vi "Экран наладки.vi"() -> ()   [LabVIEW 2011]
panel:
  in  "Закрыть окно":bool
  in  "y0":dbl
  in  "x40":dbl
  out "y0":bool[](array[boolean])
  out "y0":string[](array[string])
  out "x40":bool[](array[boolean])
  out "x40":string[](array[string])
  out "x0":bool[](array[boolean])
  out "x0":string[](array[string])
  in  "x0":dbl
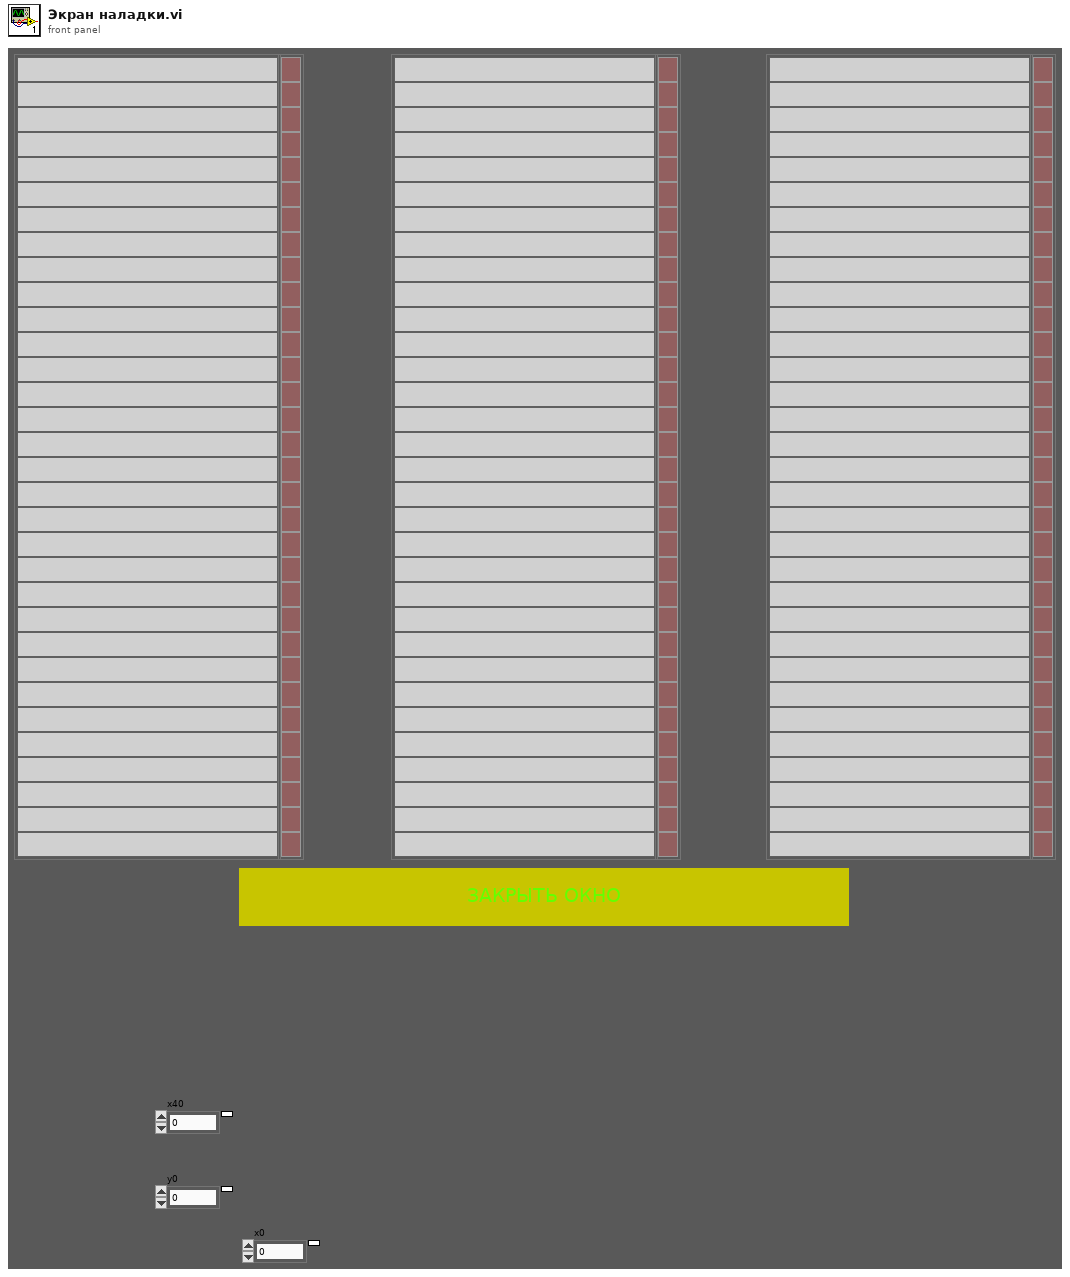
[diagram p1: front panel]
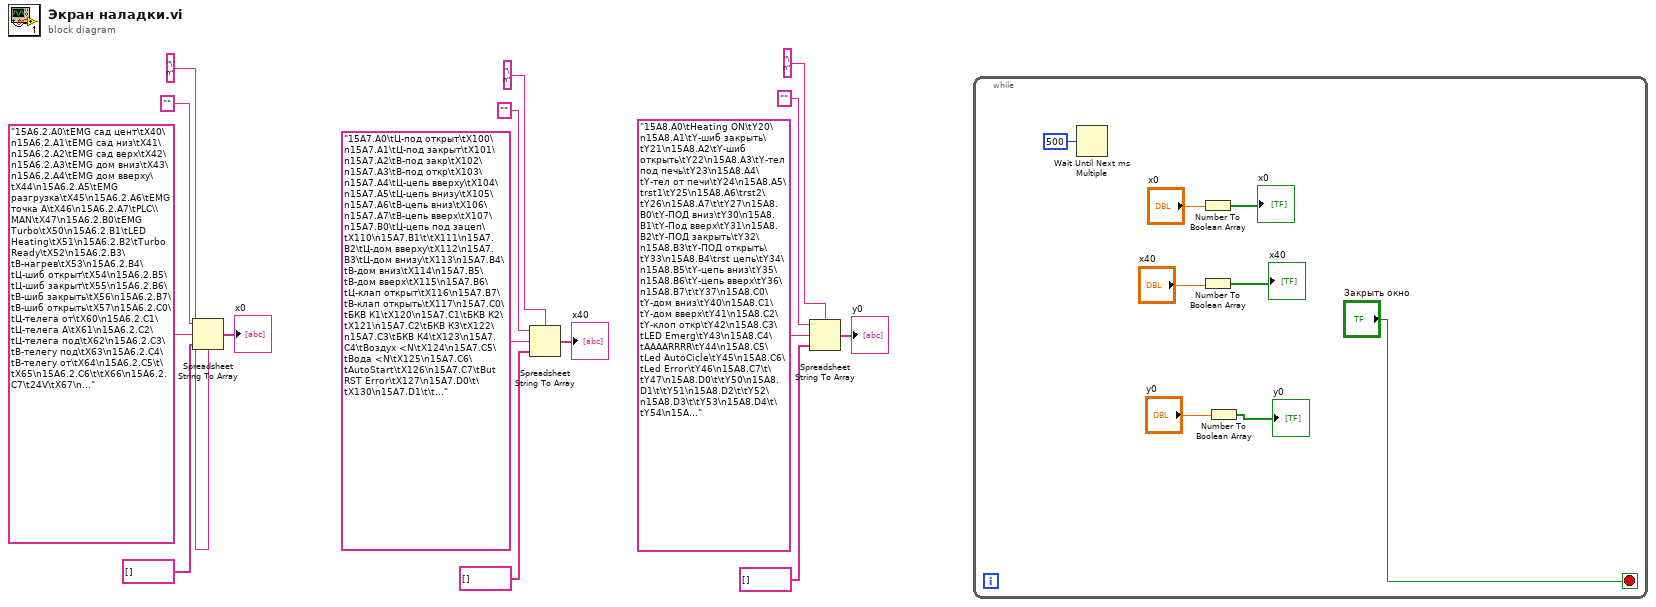
[diagram p0: block diagram]
diagram:
  n1 = Spreadsheet String To Array(delimiter (Tab)="\n", format string="", spreadsheet string="15A6.2.A0\tEMG сад цент\tX40\n15A6.2.A1\tEMG сад низ\tX41\n15A6.2.A2\tEMG сад верх\tX42\n15A6.2.A3\tEMG дом вниз\tX43\n15A6.2.A4\tEMG дом вверху\tX44\n15A6.2.A5\tEMG разгрузка\tX45\n15A6.2.A6\tEMG точка А\tX46\n15A6.2.A7\tPLC\\MAN\tX47\n15A6.2.B0\tEMG Turbo\tX50\n15A6.2.B1\tLED Heating\tX51\n15A6.2.B2\tTurbo Ready\tX52\n15A6.2.B3\tB-нагрев\tX53\n15A6.2.B4\tЦ-шиб открыт\tX54\n15A6.2.B5\tЦ-шиб закрыт\tX55\n15A6.2.B6\tВ-шиб закрыть\tX56\n15A6.2.B7\tВ-шиб открыть\tX57\n15A6.2.C0\tЦ-телега от\tX60\n15A6.2.C1\tЦ-телега А\tX61\n15A6.2.C2\tЦ-телега под\tX62\n15A6.2.C3\tВ-телегу под\tX63\n15A6.2.C4\tВ-телегу от\tX64\n15A6.2.C5\t\tX65\n15A6.2.C6\t\tX66\n15A6.2.C7\t24V\tX67\n15A6.2.D0\tЦ-под up\tX70\n15A6.2.D1\tЦ-под down\tX71\n15A6.2.D2\tВ-под вниз\tX72\n15A6.2.D3\tВ-под вверх\tX73\n15A6.2.D4\tЦ-под2 вверху\tX74\n15A6.2.D5\tЦ-под2 внизу\tX75\n15A6.2.D6\t\tX76\n15A6.2.D7\t\tX77", array type (2D Dbl)=string[] []) -> (array=→"x0":string[])
  n2 = Spreadsheet String To Array(delimiter (Tab)="\n", format string="", spreadsheet string="15A7.A0\tЦ-под открыт\tX100\n15A7.A1\tЦ-под закрыт\tX101\n15A7.A2\tВ-под закр\tX102\n15A7.A3\tВ-под откр\tX103\n15A7.A4\tЦ-цепь вверху\tX104\n15A7.A5\tЦ-цепь внизу\tX105\n15A7.A6\tВ-цепь вниз\tX106\n15A7.A7\tВ-цепь вверх\tX107\n15A7.B0\tЦ-цепь под зацеп\tX110\n15A7.B1\t\tX111\n15A7.B2\tЦ-дом вверху\tX112\n15A7.B3\tЦ-дом внизу\tX113\n15A7.B4\tВ-дом вниз\tX114\n15A7.B5\tВ-дом вверх\tX115\n15A7.B6\tЦ-клап открыт\tX116\n15A7.B7\tВ-клап открыть\tX117\n15A7.C0\tБКВ К1\tX120\n15A7.C1\tБКВ К2\tX121\n15A7.C2\tБКВ К3\tX122\n15A7.C3\tБКВ К4\tX123\n15A7.C4\tВоздух <N\tX124\n15A7.C5\tВода <N\tX125\n15A7.C6\tAutoStart\tX126\n15A7.C7\tBut RST Error\tX127\n15A7.D0\t\tX130\n15A7.D1\t\tX131\n15A7.D2\t\tX132\n15A7.D3\t\tX133\n15A7.D4\t\tX134\n15A7.D5\t\tX135\n15A7.D6\t\tX136\n15A7.D7\t\tX137", array type (2D Dbl)=string[] []) -> (array=→"x40":string[])
  n3 = Spreadsheet String To Array(delimiter (Tab)="\n", format string="", spreadsheet string="15A8.A0\tHeating ON\tY20\n15A8.A1\tY-шиб закрыть\tY21\n15A8.A2\tY-шиб открыть\tY22\n15A8.A3\tY-тел под печь\tY23\n15A8.A4\tY-тел от печи\tY24\n15A8.A5\trst1\tY25\n15A8.A6\trst2\tY26\n15A8.A7\t\tY27\n15A8.B0\tY-ПОД вниз\tY30\n15A8.B1\tY-Под вверх\tY31\n15A8.B2\tY-ПОД закрыть\tY32\n15A8.B3\tY-ПОД открыть\tY33\n15A8.B4\trst цепь\tY34\n15A8.B5\tY-цепь вниз\tY35\n15A8.B6\tY-цепь вверх\tY36\n15A8.B7\t\tY37\n15A8.C0\tY-дом вниз\tY40\n15A8.C1\tY-дом вверх\tY41\n15A8.C2\tY-клоп откр\tY42\n15A8.C3\tLED Emerg\tY43\n15A8.C4\tAAAARRRR\tY44\n15A8.C5\tLed AutoCicle\tY45\n15A8.C6\tLed Error\tY46\n15A8.C7\t\tY47\n15A8.D0\t\tY50\n15A8.D1\t\tY51\n15A8.D2\t\tY52\n15A8.D3\t\tY53\n15A8.D4\t\tY54\n15A8.D5\t\tY55\n15A8.D6\t\tY56\n15A8.D7\t\tY57\n", array type (2D Dbl)=string[] []) -> (array=→"y0":string[])
  n4 = while {
    stop <- "Закрыть окно" stop-if-true
    n5 = Wait Until Next ms Multiple(millisecond multiple=u32 500) -> ()  [unwired: 1 out]
    n6 = Number To Boolean Array(number="x0") -> (Boolean array=→"x0":bool[])
    n7 = Number To Boolean Array(number="x40") -> (Boolean array=→"x40":bool[])
    n8 = Number To Boolean Array(number="y0") -> (Boolean array=→"y0":bool[])
  }
